vi "setAO_Amp.vi"(8 "error in (no error)":errorcluster, 9 "new Amp (V)":dbl, 10 "AO Channel":i32, 11 "Channels: AO":T1={"AO amp (V)"=[0.01, 0.0, 0.0, 0.0, 0.0, 0.0, 0.0, 0.0], "AO DC (V)"=[0.0, 0.0, 0.0, 0.0, 0.0, 0.0, 0.0, 0.0], "AO f (Hz)"=[13.1, 13.0, 13.0, 13.0, 13.0, 13.0, 13.0, 13.0], "AO phi (deg)"=[0.0, 0.0, 0.0, 0.0, 0.0, 0.0, 0.0, 0.0], "function"=[enum."Sine Wave", enum."Sine Wave", enum."Sine Wave", enum."Sine Wave", enum."Sine Wave", enum."Sine Wave", enum."Sine Wave", enum."Sine Wave"]} {"AO f (Hz)" min=0.001 max=10000.0; "AO DC (V)" format="%#_6p"; "AO amp (V)" format="%#_6p"}) -> (0 "error out":errorcluster, 3 "Channels: AO":T1={"AO amp (V)"=[0.01, 0.0, 0.0, 0.0, 0.0, 0.0, 0.0, 0.0], "AO DC (V)"=[0.0, 0.0, 0.0, 0.0, 0.0, 0.0, 0.0, 0.0], "AO f (Hz)"=[13.1, 13.0, 13.0, 13.0, 13.0, 13.0, 13.0, 13.0], "AO phi (deg)"=[0.0, 0.0, 0.0, 0.0, 0.0, 0.0, 0.0, 0.0], "function"=[enum."Sine Wave", enum."Sine Wave", enum."Sine Wave", enum."Sine Wave", enum."Sine Wave", enum."Sine Wave", enum."Sine Wave", enum."Sine Wave"]} {"AO f (Hz)" min=0.001 max=10000.0; "AO DC (V)" format="%#_6p"; "AO amp (V)" format="%#_6p"})   [LabVIEW 2016]
uses:
  Typedefs/AO-cluster.ctl
  Typedefs/AO_Amp-array.ctl
  Typedefs/AO_DC-array.ctl
  Typedefs/AO_f-array.ctl
  Typedefs/AO_phi-array.ctl
  Typedefs/Function-array.ctl
  Typedefs/Function-enum.ctl
panel:
  # "0"
  # "1"
  # "2"
  # "3"
  # "4"
  # "5"
  # "6"
  # "7"
  # "0"
  # "1"
  # "2"
  # "3"
  # "4"
  # "5"
  # "6"
  # "7"
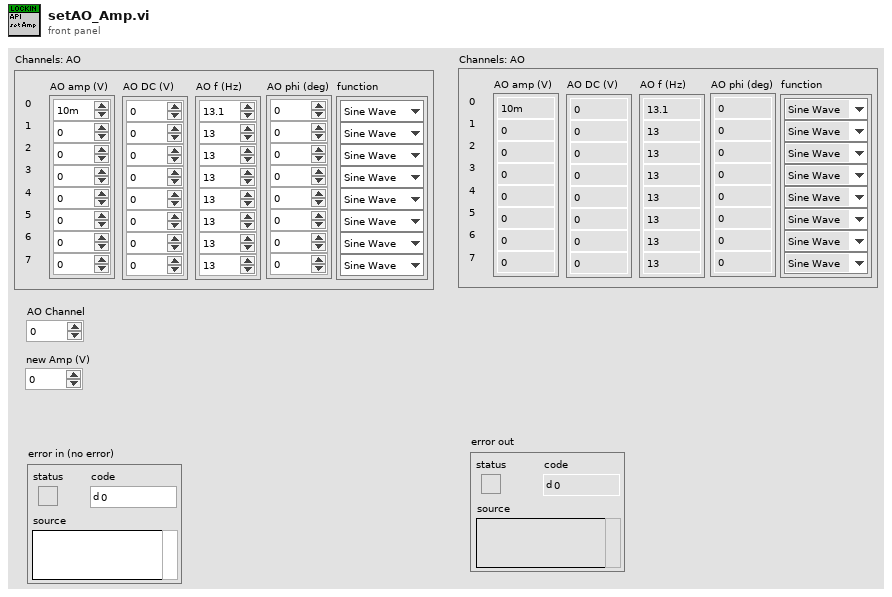
[diagram p1: front panel]
types:
  T1 = typedef "AO-cluster.ctl" = cluster{"AO amp (V)":T2, "AO DC (V)":T3, "AO f (Hz)":T4, "AO phi (deg)":T5, "function":T6}
  T2 = typedef "AO_Amp-array.ctl" = dbl[]
  T3 = typedef "AO_DC-array.ctl" = dbl[]
  T4 = typedef "AO_f-array.ctl" = dbl[]
  T5 = typedef "AO_phi-array.ctl" = dbl[]
  T6 = typedef "Function-array.ctl" = T7[]
  T7 = typedef "Function-enum.ctl" = enum16{"Sine Wave", "Triangle Wave", "Square Wave", "Sawtooth Wave"}
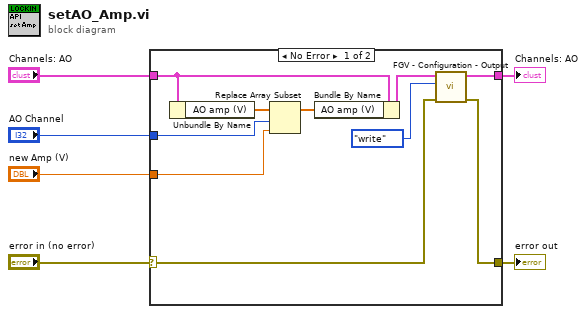
[diagram p0: block diagram]
diagram:
  n1 = case shown="No Error" "error in (no error)" {
    selector: "error in (no error)" -> [w9 w18]
    tunnel: "Channels: AO" -> [w14 w17]
    tunnel: [w10 w17] -> w5
    tunnel: "AO Channel" -> [w13 _]
    tunnel: "new Amp (V)" -> [w12 _]
    tunnel: [w8 w18] -> w1
    frame No Error {
      n2 = Unbundle By Name(w14) -> ("AO amp (V)"=w15:T2)
      n3 = Replace Array Subset(array=w15, new element=w12, index=w13) -> (w16:T2)
      n4 = Bundle By Name(cluster=w14, "AO amp (V)"=w16) -> (w11:T1)
      n5 = call "FGV - Configuration - Output.vi"("error in"=w9, "Function"=enum16{"write", "read"}."write", "Channels: AO"=w11) -> ("error out"=w8:errorcluster, "Channels: AO 2"=w10:T1)  [unwired: 3 in]
    }
    frame Error {
    }
  }
  "Channels: AO" <- w5
  "error out" <- w1
